vi "Import Data Items Nodes.vi"(8 "error in (no error)":errorcluster, 11 "Node Ptr":u64 format="%.0x") -> (0 "error out":errorcluster)   [LabVIEW 2023, in "Vires VTD System Explorer.lvlib"]
uses:
  Vires VTD System Explorer.lvlib
  Item Informations.ctl
  <vilib>/NI VeriStand/Custom Device API/Custom Device Item Info.ctl
  <vilib>/NI VeriStand/Custom Device API/Custom Device Channel.ctl
  <vilib>/NI VeriStand/Custom Device API/Custom Device Channel Type.ctl
  Data Channel Custom Property.ctl
  <vilib>/Utility/xml.llb/Read From XML File(string).vi
  <vilib>/NI VeriStand/Custom Device Tools/Custom Device Utility Library/Custom Device Utility Library.lvlib
  <vilib>/NI VeriStand/Custom Device API/Custom Device API.lvlib
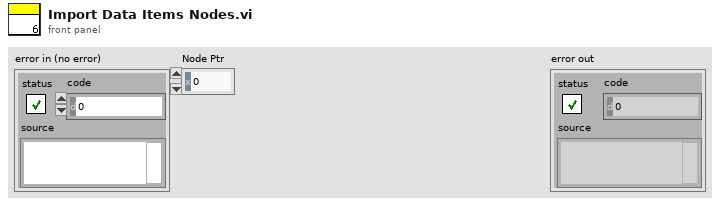
[diagram p1: front panel]
types:
  T1 = typedef "Vires VTD System Explorer.lvlib/Item Informations.ctl" = cluster{"Parents Section Names":string[], "Item Info":T2, "Channel Info":T3, "Data Channel Property":T5}
  T2 = typedef "Custom Device API.lvlib/Custom Device Item Info.ctl" = cluster{"Name":string, "Is Channel":bool, "GUID":string, "Is Waveform":bool}
  T3 = typedef "Custom Device API.lvlib/Custom Device Channel.ctl" = cluster{"Type":T4, "Units":string, "Default Value":dbl, "Faultable":bool, "Scalable":bool}
  T4 = typedef "Custom Device API.lvlib/Custom Device Channel Type.ctl" = enum16{"Input", "Output"}
  T5 = typedef "Vires VTD System Explorer.lvlib/Data Channel Custom Property.ctl" = cluster{"pkid":u32, "Signalname":string, "PlayerID":u8, "WheelID":i32}
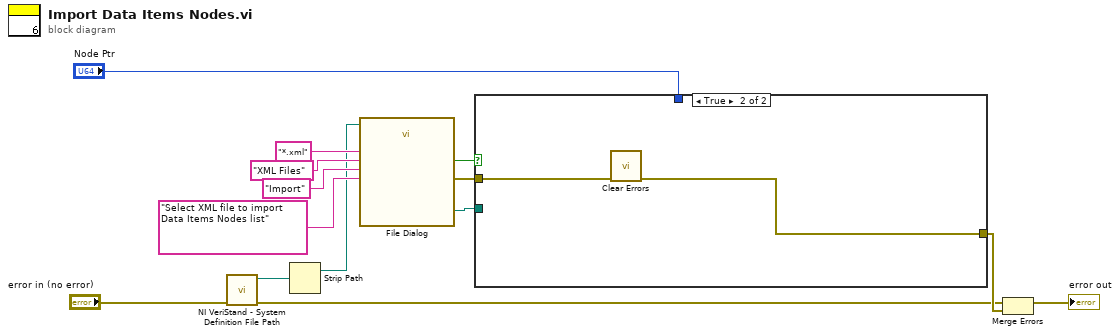
[diagram p0: block diagram]
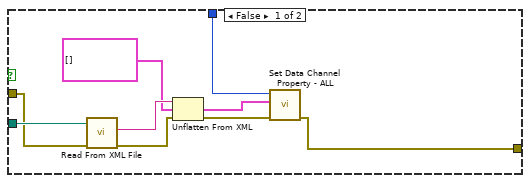
[diagram p2: hidden frame]
diagram:
  n1 = call <vilib>:"NI VeriStand - System Definition File Path.vi"("error in (no error)"="error in (no error)") -> ("error out"=w5:errorcluster, "SDF path"=w6:path)  [unwired: 9 in]
  n2 = Strip Path(path=w6) -> (stripped path=w4:path)  [unwired: 1 out]
  n3 = call "File Dialog"("start path"=w4, "prompt"="Select XML file to import Data Items Nodes list", "button label"="Import", "pattern (all files)"="*.xml", "pattern label"="XML Files") -> ("selected path"=w9:path, "cancelled"=w10:bool, "error out"=w8:errorcluster)  [unwired: 7 in, 1 out]
  n4 = case shown="True" w10 {
    tunnel: w9 -> [w23 _]
    tunnel: w8 -> [w20 w25]
    tunnel: [w15 w24] -> w7
    tunnel: "Node Ptr" -> [w17 _]
    frame False {
      n5 = call-poly <vilib>:"Read From XML File.vi"("error in (no error)"=w20, "XML File Path"=w23) -> ("error out"=w19:errorcluster, "XML Elements"=w22:string)  [unwired: 7 in, 1 out]
      n6 = Unflatten From XML(xml string=w22, type=T1[] [], error in (no error)=w19) -> (value=w18:T1[], error out=w16:errorcluster)
      n7 = call "Set Data Channel Property - ALL.vi"("error in"=w16, "Item Informations array"=w18, "Item Ref in"=w17) -> ("error out"=w15:errorcluster)  [unwired: 8 in]
    }
    frame True {
      n8 = call <vilib>:"Clear Errors.vi"("error in (no error)"=w25) -> ("error out"=w24:errorcluster)  [unwired: 5 in, 1 out]
    }
  }
  n9 = Merge Errors(w5, w7) -> (→"error out":errorcluster)
